vi "Unwrap Phase.vi"(10 "phase unit":i32(ring) items=["radian in, radian out", "radian in, degree out", "degree in, degree out", "degree in, radian out"], 11 "Phase":dbl[](array[numeric])) -> (0 "error":i32, 3 "Unwrapped Phase":dbl[](array[numeric]))   [LabVIEW 2010, in "NI_AALPro.lvlib"]
doc: "Unwraps the <B>Phase</B> array by eliminating discontinuities whose absolute values exceed either pi or 180, depending on the units you specify in <B>phase unit</B>."
uses:
  NI_AALPro.lvlib
  lvanlys.dll
panel:
  # "Unwrap Phase"
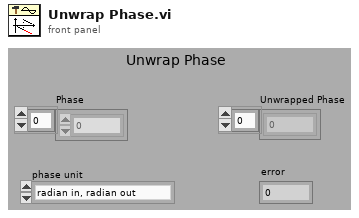
[diagram p1: front panel]
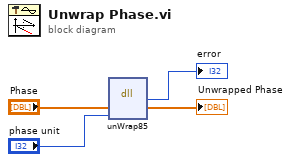
[diagram p0: block diagram]
diagram:
  n1 = dll-call lib="C:/Program Files/National Instruments/LabVIEW 2010/resource/lvanlys.*" fn="unWrap85"("Phase"="Phase", "phase unit"="phase unit") -> ("return type"=→"error":i32, "Phase"=→"Unwrapped Phase":dbl[])  [unwired: 4 in, 2 out]
